vi "Pfeiffer Vacuum OnTool Operating adjustment.vi"(8 "error in (no error)":errorcluster, 9 "PV OnTool Op adjustment - Cluster":T1={"Parameter"=0, "Parameter\nread only<->describe"=FALSE, "off<->on"=TRUE, "Rotation speed set value\nin rot. speed setting\noperations [%]"=100.0, "Operations mode pump"=0} {"Operations mode pump" items=[" Rotations speed", " Final Speed operation", " Loadlock (Softpumping)", " Idle"]; "Rotation speed set value\nin rot. speed setting\noperations [%]" min=15.0 max=100.0 step=0.1 format="%.2f"; "Parameter" items=[" Pumping station", " Operations mode pump", " Rotation speed set value in rot. speed setting operations", " Set rotation speed BkP [Hz] (read only)", " Actual rotation speed BkP [Hz] (read only)", " Power supply version"]}, 10 "Adress of unit":u16=1 min=1 max=999 step=1, 11 "COM Port Name in":refnum<visa-resource-name>="COM1") -> (0 "error out":errorcluster, 1 "response (data)":string)   [LabVIEW 2021]
doc: "This VI is an example of how to use the Pfeiffer Vacuum subVIs programmatically. This VI first initializes the instrument, takes measurements, then closes the instrument."
uses:
  <instrlib>/Pfeiffer Vacuum/Public/OnTool/PV OnTool Op adjustment - Cluster.ctl
  <instrlib>/Pfeiffer Vacuum/Pfeiffer Vacuum.lvlib
panel:
  # "Pumping station                   :\n Power supply version         :"
  # "<----------\n off\n 3 phases"
  # "---------->     \non \n1 phases"
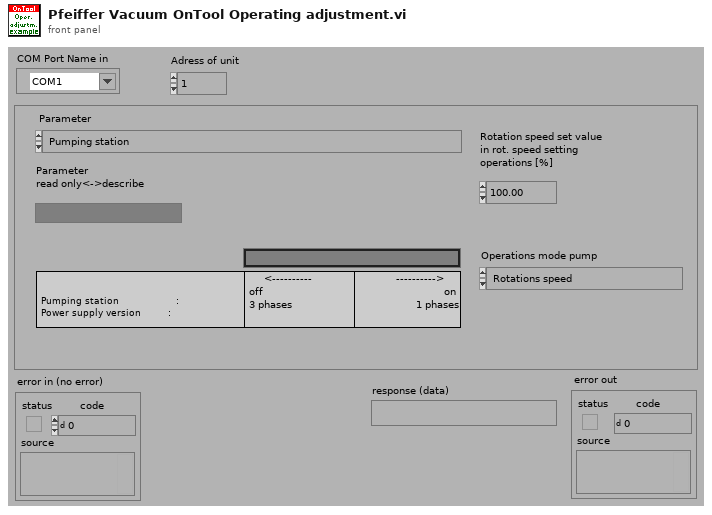
[diagram p1: front panel]
types:
  T1 = typedef "Pfeiffer Vacuum.lvlib/PV OnTool Op adjustment - Cluster.ctl" = cluster{"Parameter":u16, "Parameter\nread only<->describe":bool, "off<->on":bool, "Rotation speed set value\nin rot. speed setting\noperations [%]":dbl, "Operations mode pump":u16}
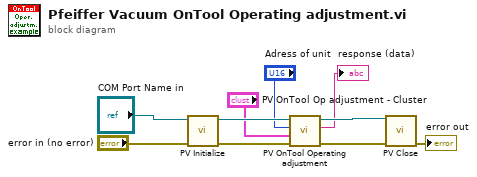
[diagram p0: block diagram]
diagram:
  n1 = call <instrlib>:"PV Initialize.vi"("error in (no error)"="error in (no error)", "VISA session in"="COM Port Name in") -> ("error out"=w8:errorcluster, "VISA session out"=w6:refnum<visa-resource-name>)  [unwired: 8 in]
  n2 = call <instrlib>:"PV OnTool Operating adjustment.vi"("error in (no error)"=w8, "PV OnTool Op adjustment - Cluster"="PV OnTool Op adjustment - Cluster", "Adress of unit"="Adress of unit", "VISA session"=w6) -> ("error out"=w7:errorcluster, "response (data)"=→"response (data)":string, "dup VISA session"=w5:refnum<visa-resource-name>)  [unwired: 5 in]
  n3 = call <instrlib>:"PV Close.vi"("VISA session"=w5, "error in (no error)"=w7) -> ("error out"=→"error out":errorcluster)  [unwired: 13 in]
